vi "FV-resample-split_NanoVNA.vi"(7 "min Frequency":dbl, 10 "NanoVNA":T1) -> (2 "output cluster":T1)   [LabVIEW 2020, in "FV-file_viewer.lvlib"]
uses:
  FV-file_viewer.lvlib
  record_file_handler/VFH-file_cluster-NanoVNA.ctl
  record_file_handler/VFH-VNA_File_Handler.lvlib
panel:
  out "Frequency":dbl[](array[numeric])
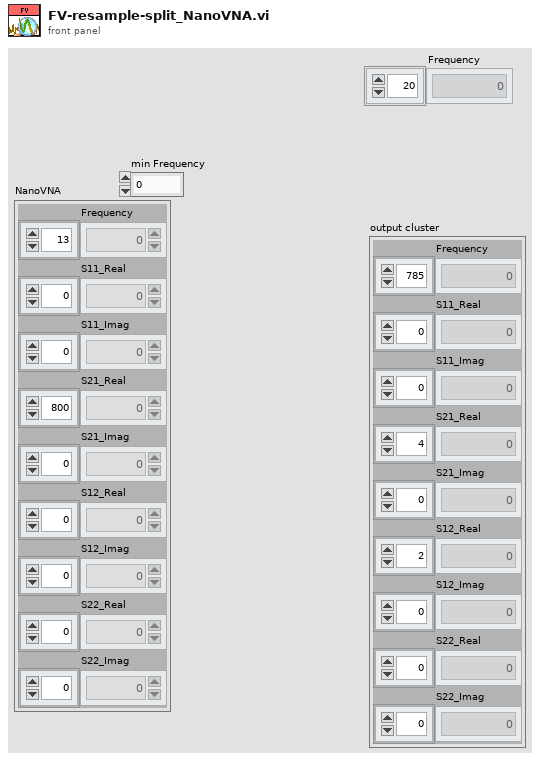
[diagram p1: front panel]
types:
  T1 = typedef "VFH-VNA_File_Handler.lvlib/VFH-file_cluster-NanoVNA.ctl" = cluster{"Frequency":dbl[], "S11_Real":dbl[], "S11_Imag":dbl[], "S21_Real":dbl[], "S21_Imag":dbl[], "S12_Real":dbl[], "S12_Imag":dbl[], "S22_Real":dbl[], "S22_Imag":dbl[]}
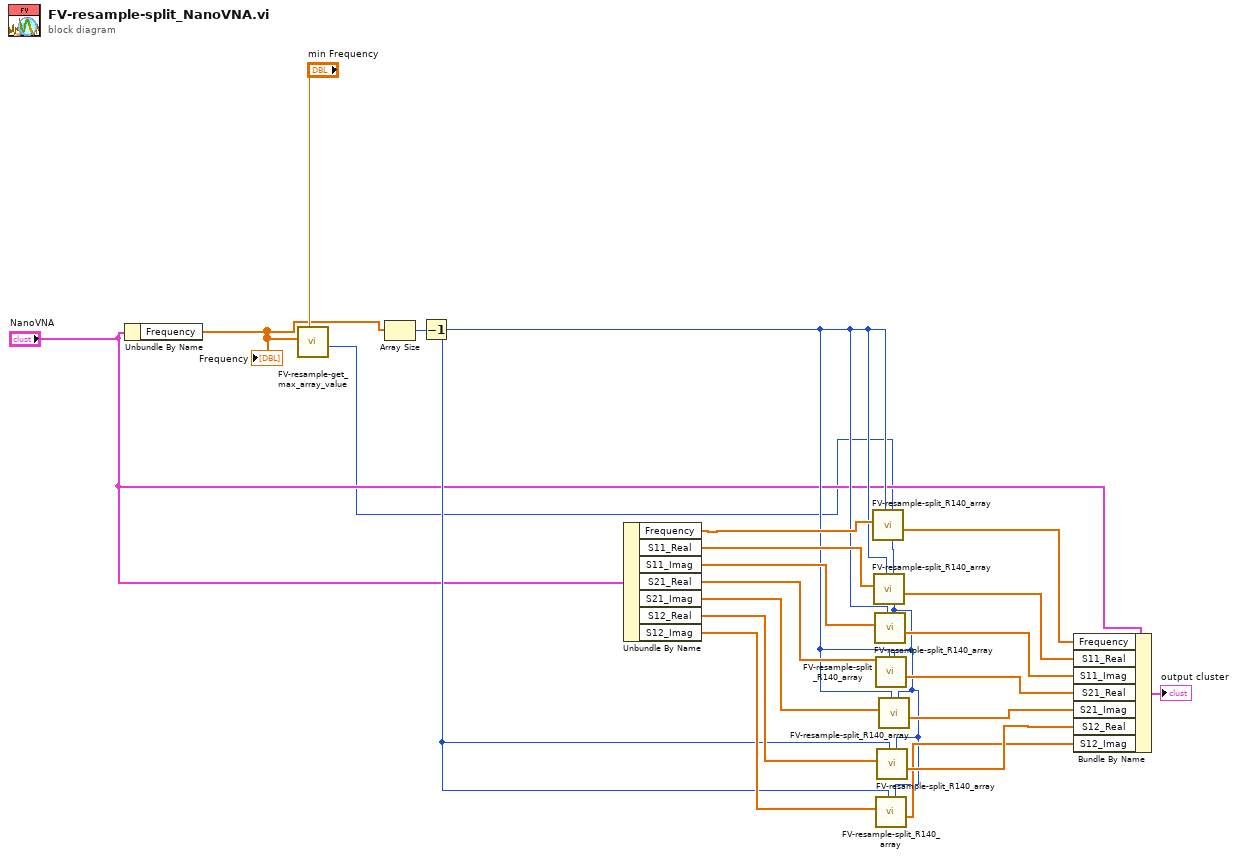
[diagram p0: block diagram]
diagram:
  n1 = Unbundle By Name("NanoVNA") -> ("Frequency"=w2:dbl[])
  "Frequency" <- w2
  n2 = call "FV-resample-get_max_array_value.vi"("max Frequency"="min Frequency", "Frequency array"=w2) -> ("Position"=w1:i32)  [unwired: 8 in, 1 out]
  n3 = Array Size(array=w2) -> (size(s)=w20:i32)
  n4 = Decrement(x=w20) -> (x-1=w5:i32)
  n5 = Unbundle By Name("NanoVNA") -> ("Frequency"=w19:dbl[], "S11_Real"=w18:dbl[], "S11_Imag"=w17:dbl[], "S21_Real"=w16:dbl[], "S21_Imag"=w15:dbl[], "S12_Real"=w14:dbl[], "S12_Imag"=w13:dbl[])
  n6 = call "FV-resample-split_R140_array.vi"("Mid split"=w1, "First split"=w5, "double array"=w19) -> ("second subarray"=w12:dbl[])  [unwired: 7 in, 1 out]
  n7 = call "FV-resample-split_R140_array.vi"("Mid split"=w1, "First split"=w5, "double array"=w18) -> ("second subarray"=w11:dbl[])  [unwired: 7 in, 1 out]
  n8 = call "FV-resample-split_R140_array.vi"("Mid split"=w1, "First split"=w5, "double array"=w17) -> ("second subarray"=w10:dbl[])  [unwired: 7 in, 1 out]
  n9 = call "FV-resample-split_R140_array.vi"("Mid split"=w1, "First split"=w5, "double array"=w16) -> ("second subarray"=w9:dbl[])  [unwired: 7 in, 1 out]
  n10 = call "FV-resample-split_R140_array.vi"("Mid split"=w1, "First split"=w5, "double array"=w13) -> ("second subarray"=w6:dbl[])  [unwired: 7 in, 1 out]
  n11 = call "FV-resample-split_R140_array.vi"("Mid split"=w1, "First split"=w5, "double array"=w14) -> ("second subarray"=w7:dbl[])  [unwired: 7 in, 1 out]
  n12 = call "FV-resample-split_R140_array.vi"("Mid split"=w1, "First split"=w5, "double array"=w15) -> ("second subarray"=w8:dbl[])  [unwired: 7 in, 1 out]
  n13 = Bundle By Name(cluster="NanoVNA", "Frequency"=w12, "S11_Real"=w11, "S11_Imag"=w10, "S21_Real"=w9, "S21_Imag"=w8, "S12_Real"=w7, "S12_Imag"=w6) -> (→"output cluster":T1)
